vi "Assert No Error.vi"(7 "Status":T1=enum."Failed", 8 "error In":errorcluster, 10 "Assert error":errorcluster, 11 "LUnit Test Case In":refnum<class "LUnit Test Case.lvclass">) -> (0 "error out":errorcluster, 3 "LUnit Test Case Out":refnum<class "LUnit Test Case.lvclass">)   [LabVIEW 2020, in "LUnit Test Case.lvclass"]
doc: "Generates a fail result for the calling test method if the inputs contains an error with status \"True\". A description may be provided to the result."
uses:
  LUnit Test Case.lvclass
  Core/Result/Status.ctl
  Core/Result/Type.ctl
  Core/Result/Result.ctl
  LUnit Test Case.lvclass/LUnit Test Case.ctl
  Core/Result/Result.lvlib
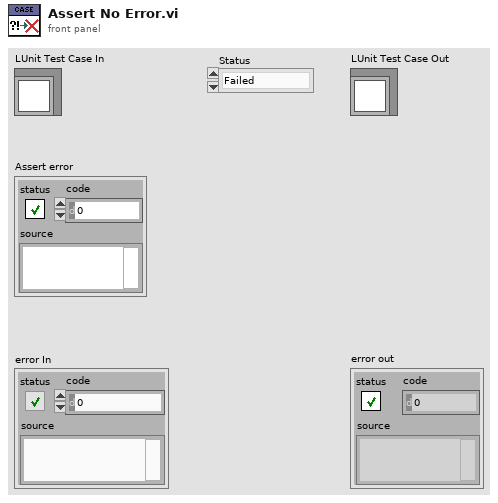
[diagram p1: front panel]
types:
  T1 = typedef "Result.lvlib/Status.ctl" = enum16{"", "Passed", "Failed", "Error", "Skipped", "Setup Error", "Broken", "Teardown Error"}
  T2 = typedef "Result.lvlib/Type.ctl" = enum16{"Test Case", "Test Suite", "Test Run", "Pass", "Fail", "Skip", "Pass if", "Fail if", "Pass if Error", "Fail if Error", "Pass if Equal", "Fail if Equal"}
  T3 = typedef "Result.lvlib/Result.ctl" = cluster{"Name":string, "Message":string, "Description":string, "Status":T1, "Result Type":T2, "Execution Time":dbl}
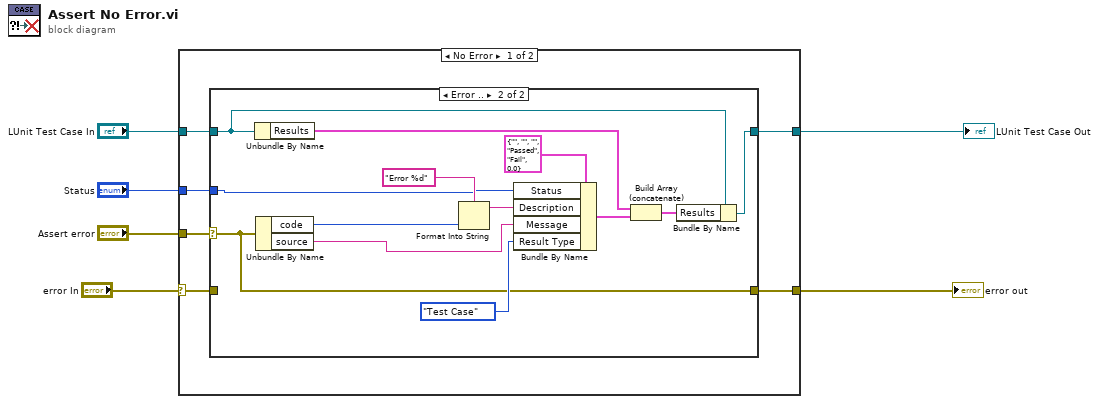
[diagram p0: block diagram]
diagram:
  n1 = case shown="No Error" "error In" {
    selector: "error In" -> [w7 w29]
    tunnel: "Assert error" -> [w12 _]
    tunnel: "LUnit Test Case In" -> [w11 w28]
    tunnel: [w10 w28] -> w4
    tunnel: "Status" -> [w9 _]
    tunnel: [w8 w29] -> w2
    frame No Error {
      n2 = case shown="Error .." w12 {
        selector: w12 -> [_ w17]
        tunnel: w11 -> [w14 w27]
        tunnel: [w14 w26] -> w10
        tunnel: w9 -> [_ w15]
        tunnel: [w13 w17] -> w8
        tunnel: w7 -> [w13 _]
        frame No Error {
        }
        frame Error {
          n3 = Unbundle By Name(w27) -> ("Results"=w21:T3[])
          n4 = Unbundle By Name(w17) -> ("code"=w23:i32, "source"=w16:string)
          n5 = Format Into String(format string="Error %d", w23) -> (resulting string=w25:string)  [unwired: 2 in, 1 out]
          n6 = Bundle By Name(cluster=T3 {"Name"="", "Message"="", "Description"="", "Status"=enum."Passed", "Result Type"=enum."Fail", "Execution Time"=0.0} ("Temporary Assertion Result"), "Status"=w15, "Description"=w25, "Message"=w16, "Result Type"=Type."Test Case") -> (w20:T3)
          n7 = Build Array (concatenate)(w21, w20) -> (w22:T3[])
          n8 = Bundle By Name(cluster=w27, "Results"=w22) -> (w26:refnum<class "LUnit Test Case.lvclass">)
        }
      }
    }
    frame Error {
    }
  }
  "error out" <- w2
  "LUnit Test Case Out" <- w4
